vi "test_HostWrite__Host.vi"() -> ()   [LabVIEW 2014]
uses:
  <vilib>/WebDAVClient/Advanced/Put File.vi
  <vilib>/WebDAVClient/NI_WebDAV.lvlib
panel:
  out "x = 0? 2":bool
  out "x = 0?":bool
  out "comm_myrio":bool
  in  "String":string
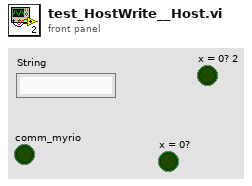
[diagram p1: front panel]
types:
  T1 = typedef "NI_WebDAV.lvlib/SessionHandle.ctl" = refnum<k1>
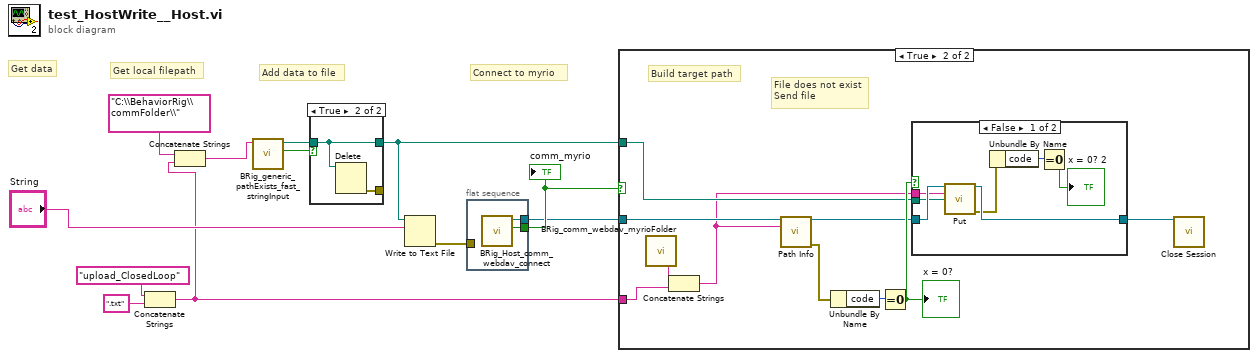
[diagram p0: block diagram]
diagram:
  # "Connect to myrio"
  # "Add data to file"
  # "Get local filepath"
  # "Get data"
  n1 = Concatenate Strings("upload_ClosedLoop" ("string"), ".txt" ("string")) -> (w2:string)
  n2 = Concatenate Strings("C:\\BehaviorRig\\commFolder\\", w2) -> (w1:string)
  n3 = call "BRig_generic_pathExists_fast_stringInput.vi"("input_filePath"=w1) -> ("output_Iexist"=w12:bool, "output_filePath"=w11:path)  [unwired: 8 in, 1 out]
  n4 = case shown="True" w12 {
    tunnel: w11 -> [w13 w14]
    tunnel: [_ w15] -> _
    tunnel: [w13 w14] -> w6
    frame False {
    }
    frame True {
      n5 = Delete(path (use dialog)=w14) -> (error out=w15:errorcluster)  [unwired: 4 in, 2 out]
    }
  }
  n6 = Write to Text File(file (use dialog)=w6, text="String") -> (error out=w9:errorcluster)  [unwired: 2 in, 2 out]
  n7 = flat-sequence {
    tunnel: w9 -> [_]
    tunnel: [w17] -> w8
    tunnel: [w16] -> w7
    frame #0 {
      n8 = call "BRig_Host_comm_webdav_connect.vi"() -> ("output_Iconnected"=w17:bool, "output_hSession"=w16:T1)  [unwired: 9 in, 1 out]
    }
  }
  n9 = case shown="True" w8 {
    tunnel: w7 -> [_ w25]
    tunnel: w6 -> [_ w19]
    tunnel: w2 -> [_ w26]
    frame False {
    }
    frame True {
      # "File does not exist\nSend file"
      # "Build target path"
      n10 = call "BRig_comm_webdav_myrioFolder.vi"() -> ("output_myrioFolder"=w27:string)  [unwired: 11 in]
      n11 = Concatenate Strings(w27, w26) -> (w18:string)
      n12 = call <vilib>:"Path Info.vi"("session handle"=w25, "relative uri"=w18) -> ("session handle out"=w21:T1, "error out"=w23:errorcluster)  [unwired: 10 in, 2 out]
      n13 = Unbundle By Name(w23) -> ("code"=w24:i32)
      n14 = Equal To 0?(x=w24) -> (x = 0?=w22:bool)
      "x = 0?" <- w22
      n15 = case shown="False" w22 {
        tunnel: w21 -> [w34 w35]
        tunnel: [w33 w35] -> w20
        tunnel: w19 -> [w32 _]
        tunnel: w18 -> [w31 _]
        frame False {
          n16 = call-poly <vilib>:"Put.vi"("session handle"=w34, "relative uri"=w31, "local file path"=w32) -> ("session handle out"=w33:T1, "error out"=w29:errorcluster)  [unwired: 10 in, 1 out]
          n17 = Unbundle By Name(w29) -> ("code"=w30:i32)
          n18 = Equal To 0?(x=w30) -> (x = 0?=→"x = 0? 2":bool)
        }
        frame True {
        }
      }
      n19 = call <vilib>:"Close Session.vi"("session handle"=w20) -> ()  [unwired: 14 in, 1 out]
    }
  }
  "comm_myrio" <- w8
